vi "chart axis set num font.vi"(8 "error in (no error)":errorcluster, 10 "font":T1, 11 "axis":u32) -> (0 "error out":errorcluster, 2 "font out":T1)   [LabVIEW 8.6]
doc: "void chart_axis_set_num_font(lxw_chart_axis axis, lxw_chart_font *font);"
uses:
  pending_lvxlsxwriter/xlsxwriter.dll
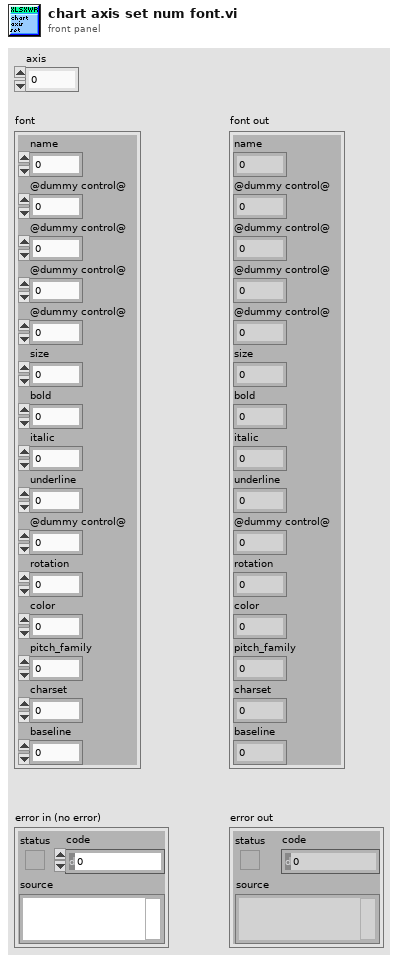
[diagram p1: front panel]
types:
  T1 = cluster{"name":u32, "@dummy control@":i8, "@dummy control@":i8, "@dummy control@":i8, "@dummy control@":i8, "size":dbl, "bold":u8, "italic":u8, "underline":u8, "@dummy control@":i8, "rotation":i32, "color":u32, "pitch_family":u8, "charset":u8, "baseline":i8}
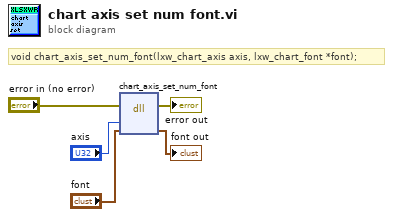
[diagram p0: block diagram]
diagram:
  # "void chart_axis_set_num_font(lxw_chart_axis axis, lxw_chart_font *font);"
  n1 = dll-call lib="C:/Users/WDAGUtilityAccount/Desktop/pending_lvxlsxwriter/xlsxwriter.*" fn="chart_axis_set_num_font"(error in="error in (no error)", "axis"="axis", "font"="font") -> (error out=→"error out":errorcluster, "font"=→"font out":T1)  [unwired: 4 in, 1 out]
